vi "Polynomials Composition (CDB).vi"(8 "threshold type":T1 items=["Absolute Value", "Relative Value"], 9 "threshold":dbl, 10 "Q(x)":cdb[](array[numeric]), 11 "P(x)":cdb[](array[numeric])) -> (0 "error":i32, 3 "P(Q(x))":cdb[](array[numeric]))   [LabVIEW 2014, in "NI_AALPro.lvlib"]
doc: "Computes the composition of polynomials <B>P(x)</B> and <B>Q(x)</B>. The data types you wire to the <B>P(x)</B> and <B>Q(x)</B> inputs determine the polymorphic instance to use."
uses:
  NI_AALPro.lvlib
  Remove Zero Threshold Type.ctl
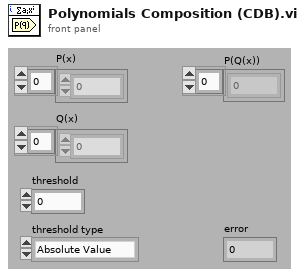
[diagram p1: front panel]
types:
  T1 = typedef "NI_AALPro.lvlib/Remove Zero Threshold Type.ctl" = u16
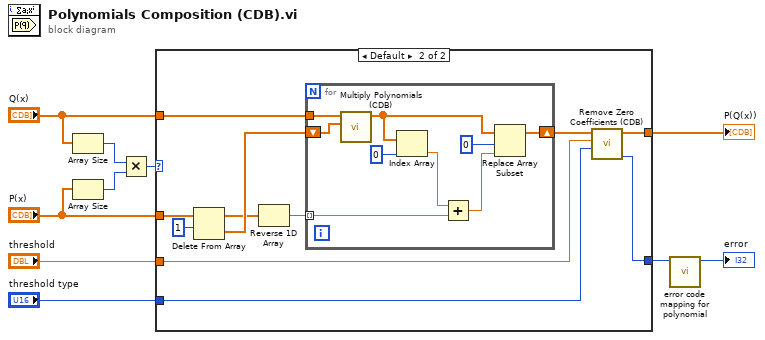
[diagram p0: block diagram]
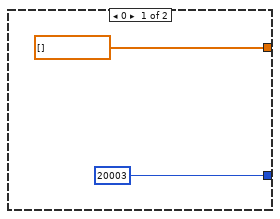
[diagram p2: hidden frame]
diagram:
  n1 = Array Size(array="Q(x)") -> (size(s)=w7:i32)
  n2 = Array Size(array="P(x)") -> (size(s)=w6:i32)
  n3 = Multiply(x=w7, y=w6) -> (x*y=w5:i32)
  n4 = case shown="Default" w5 {
    tunnel: "P(x)" -> [_ w19]
    tunnel: "Q(x)" -> [_ w22]
    tunnel: [cdb[] [] ("CDB") w20] -> w10
    tunnel: [20003 ("empty array") w15] -> w4
    tunnel: "threshold" -> [_ w14]
    tunnel: "threshold type" -> [_ w13]
    frame 0 {
    }
    frame Default {
      n5 = Delete From Array(array=w19, length=1) -> (deleted portion=w18:cdb[], array with subset deleted=w17:cdb[])  [unwired: 1 in]
      n6 = Reverse 1D Array(array=w17) -> (reversed array=w16:cdb[])
      n7 = for {
        tunnel: w16 -> [w31] mode=indexing
        tunnel: w22 -> [w25]
        shift-right: [w29] -> w21
        shift-left: w18 -> [w24]
        n8 = call "Multiply Polynomials (CDB).vi"("Q(x)"=w24, "P(x)"=w25) -> ("P(x)*Q(x)"=w26:cdb[])  [unwired: 8 in, 1 out]
        n9 = Index Array(array=w26, index=0) -> (element=w32:cdb)
        n10 = Add(x=w32, y=w31) -> (x+y=w30:cdb)
        n11 = Replace Array Subset(array=w26, new element=w30, index=0) -> (w29:cdb[])
      }
      n12 = call "Remove Zero Coefficients (CDB).vi"("threshold type"=w13, "threshold"=w14, "P(x) In"=w21) -> ("error"=w15:i32, "P(x) Out"=w20:cdb[])  [unwired: 6 in, 1 out]
    }
  }
  "P(Q(x))" <- w10
  n13 = call "error code mapping for polynomial.vi"("error in"=w4) -> ("error out"=→"error":i32)  [unwired: 10 in]
